vi "load background image.vi"(8 "error in (no error)":errorcluster, 11 "Cascade in":refnum<class "Cascade.lvclass">) -> (0 "error out":errorcluster, 3 "Cascade out":refnum<class "Cascade.lvclass">)   [LabVIEW 2012, in "Cascade.lvclass"]
uses:
  Cascade.lvclass
  Cascade.lvclass/Cascade.ctl
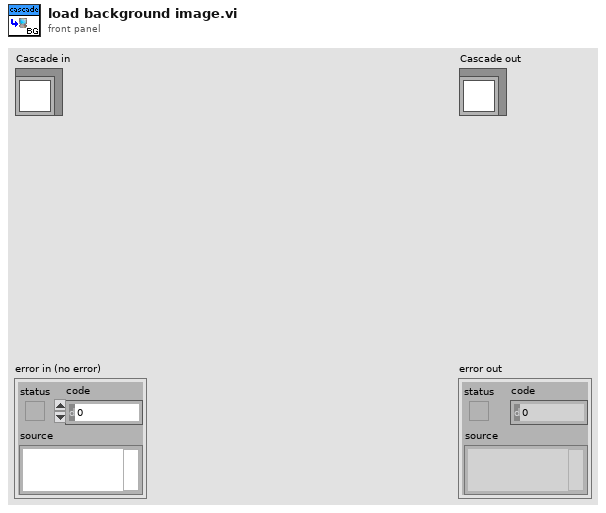
[diagram p1: front panel]
types:
  T1 = typedef "IMAQ Image.ctl" = refnum<image>
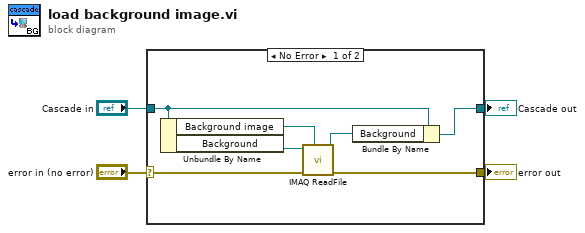
[diagram p0: block diagram]
diagram:
  n1 = case shown="No Error" "error in (no error)" {
    selector: "error in (no error)" -> [w9 w13]
    tunnel: [w8 w13] -> w3
    tunnel: [w6 w12] -> w1
    tunnel: "Cascade in" -> [w7 w12]
    frame No Error {
      n2 = Unbundle By Name(w7) -> ("Background image"=w11:path, "Background"=w10:T1)
      n3 = call "IMAQ ReadFile"("File Path"=w11, "error in (no error)"=w9, "Image"=w10) -> ("error out"=w8:errorcluster, "Image Out"=w5:T1)  [unwired: 4 in, 3 out]
      n4 = Bundle By Name(cluster=w7, "Background"=w5) -> (w6:refnum<class "Cascade.lvclass">)
    }
    frame Error {
    }
  }
  "error out" <- w3
  "Cascade out" <- w1
